vi "strain-offset_fgv.vi"(7 "cmd":enum16{"ini", "write", "read"}(ring), 8 "error in (no error)":errorcluster caption="error in", 11 "data":waveform(dbl)[](array[waveform])) -> (0 "error out":errorcluster, 3 "Strain_offset_data":waveform(dbl)[](array[waveform]))   [LabVIEW 2016]
uses:
  <vilib>/Analysis/baseanly.llb/Mean (DBL).vi
  <vilib>/Analysis/NI_AALBase.lvlib
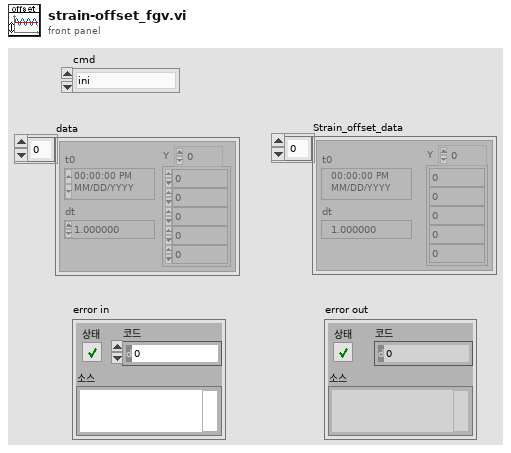
[diagram p1: front panel]
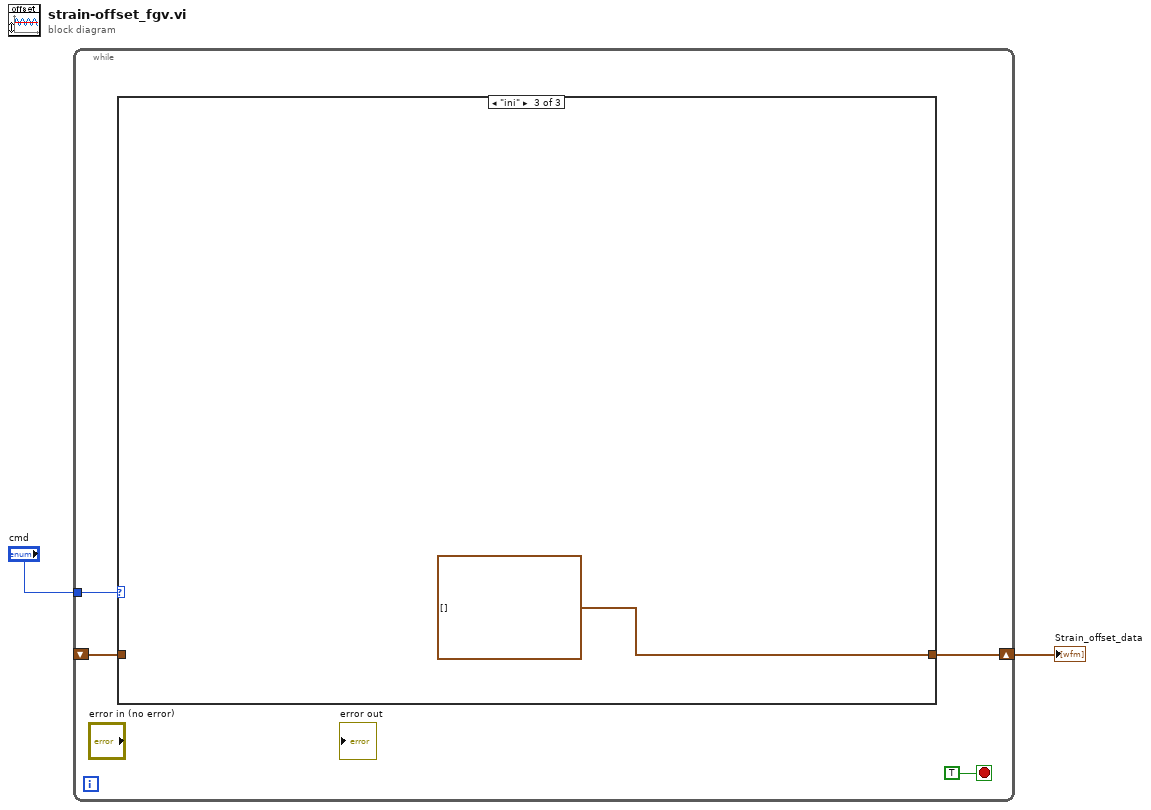
[diagram p0: block diagram]
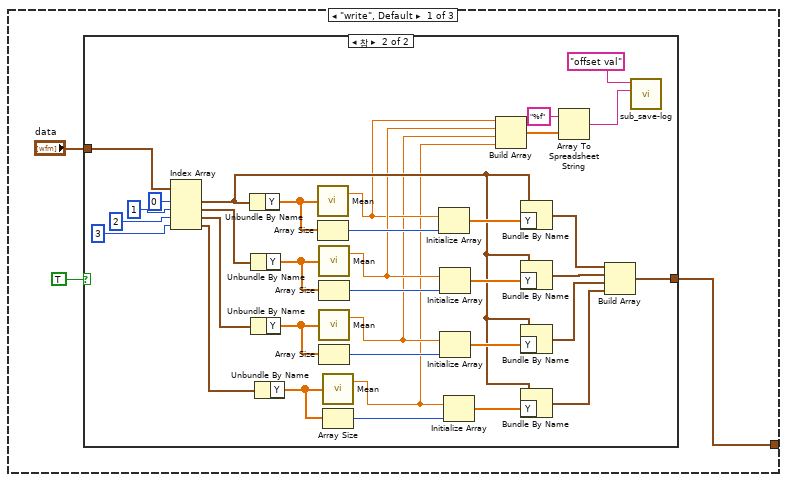
[diagram p2: hidden frame]
diagram:
  n1 = while {
    tunnel: "cmd" -> [w5]
    shift-right: [w4] -> w1
    shift-left: _ -> [w3]
    stop <- TRUE stop-if-true
    n2 = case shown="\"ini\"" w5 {
      tunnel: [w7 w45 waveform(dbl)[] [] ("data")] -> w4
      tunnel: w3 -> [_ w45 _]
      frame "write", Default {
        n3 = case shown="참" TRUE {
          tunnel: "data" -> [w10 w44]
          tunnel: [w10 w19] -> w7
          frame False {
          }
          frame True {
            n4 = Index Array(array=w44, index #1=0 ("인덱스"), index #2=1 ("인덱스"), index #3=2 ("인덱스"), index #4=3 ("인덱스")) -> (element #1=w24:waveform(dbl), element #2=w31:waveform(dbl), element #3=w30:waveform(dbl), element #4=w29:waveform(dbl))
            n5 = Unbundle By Name(w24) -> ("Y"=w39:dbl[])
            n6 = Unbundle By Name(w31) -> ("Y"=w37:dbl[])
            n7 = Unbundle By Name(w30) -> ("Y"=w35:dbl[])
            n8 = Unbundle By Name(w29) -> ("Y"=w33:dbl[])
            n9 = call-poly <vilib>:"Mean.vi"("X"=w39) -> ("mean"=w17:dbl)  [unwired: 1 out]
            n10 = Array Size(array=w39) -> (size(s)=w38:i32)
            n11 = call-poly <vilib>:"Mean.vi"("X"=w37) -> ("mean"=w18:dbl)  [unwired: 1 out]
            n12 = Array Size(array=w37) -> (size(s)=w36:i32)
            n13 = call-poly <vilib>:"Mean.vi"("X"=w35) -> ("mean"=w16:dbl)  [unwired: 1 out]
            n14 = Array Size(array=w35) -> (size(s)=w34:i32)
            n15 = call-poly <vilib>:"Mean.vi"("X"=w33) -> ("mean"=w15:dbl)  [unwired: 1 out]
            n16 = Array Size(array=w33) -> (size(s)=w32:i32)
            n17 = Initialize Array(w17, w38) -> (w28:dbl[])
            n18 = Initialize Array(w18, w36) -> (w27:dbl[])
            n19 = Initialize Array(w16, w34) -> (w26:dbl[])
            n20 = Initialize Array(w15, w32) -> (w25:dbl[])
            n21 = Build Array(w17, w18, w16, w15) -> (w14:dbl[])
            n22 = Bundle By Name(cluster=w24, "Y"=w28) -> (w20:waveform(dbl))
            n23 = Bundle By Name(cluster=w24, "Y"=w27) -> (w21:waveform(dbl))
            n24 = Bundle By Name(cluster=w24, "Y"=w26) -> (w22:waveform(dbl))
            n25 = Bundle By Name(cluster=w24, "Y"=w25) -> (w23:waveform(dbl))
            n26 = Array To Spreadsheet String(array=w14, 3:"%f" ("포맷 문자열")) -> (spreadsheet string=w13:string)  [unwired: 1 in]
            n27 = Build Array(w20, w21, w22, w23) -> (w19:waveform(dbl)[])
            n28 = call "sub_save-log.vi"("data"=w13, "title"="offset val") -> ()  [unwired: 9 in, 1 out]
          }
        }
      }
      frame "read" {
      }
      frame "ini" {
      }
    }
  }
  "Strain_offset_data" <- w1
